vi "Combine Frame Data.vi"(7 "Block Diagram":T3, 10 "Frames-Owners":T5(array[cluster]), 11 "Frames Array":T4(array[cluster])) -> (3 "Frame Data":T2(array[cluster]))   [LabVIEW 2026]
doc: "This VI takes in the array of Frames and the array mapping the frames to their owners and combines them, returning an array of clusters that contain the data from the frame array and the owner uid for each frame."
uses:
  <vilib>/picture/picture.llb/imagedata.ctl
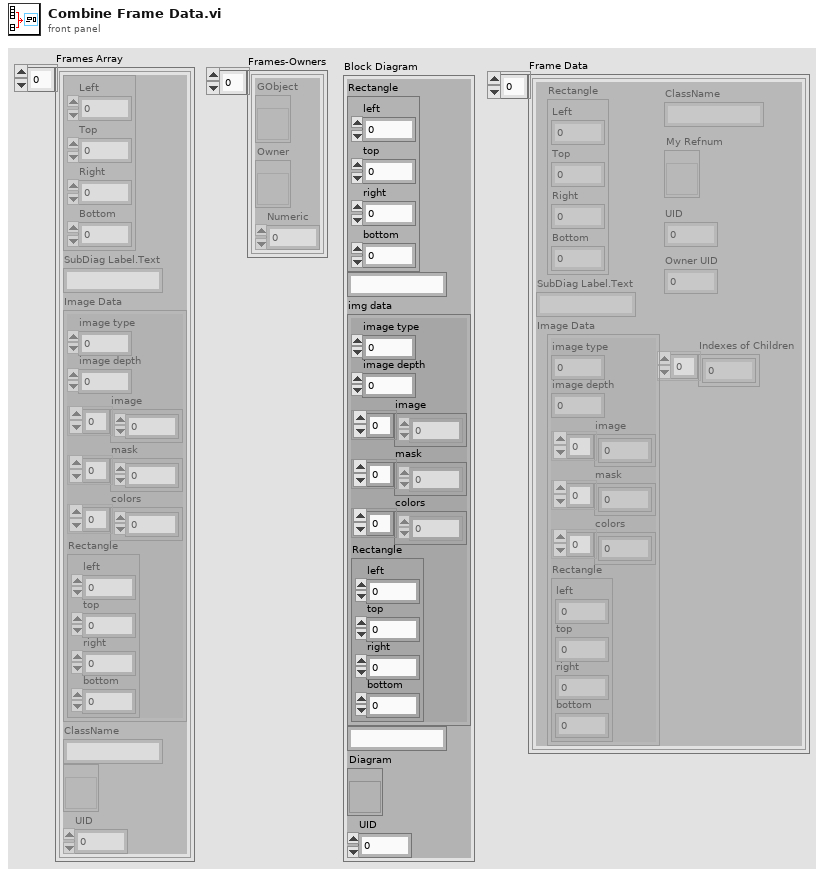
[diagram p1: front panel]
types:
  T1 = typedef "imagedata.ctl" = cluster{"image type":i32, "image depth":i32, "image":u8[], "mask":u8[], "colors":u32[], "Rectangle":cluster{"left":i16, "top":i16, "right":i16, "bottom":i16}}
  T2 = cluster{"Rectangle":cluster{"Left":i32, "Top":i32, "Right":u32, "Bottom":u32}, "SubDiag Label.Text":string, "Image Data":T1, "ClassName":string, "My Refnum":refnum<vi>, "UID":i32, "Owner UID":i32, "Indexes of Children":i32[]}[]
  T3 = cluster{"Rectangle":cluster{"left":i16, "top":i16, "right":i16, "bottom":i16}, string, "img data":T1, string, "Diagram":refnum<vi>, "UID":i32}
  T4 = cluster{cluster{"Left":i32, "Top":i32, "Right":u32, "Bottom":u32}, "SubDiag Label.Text":string, "Image Data":T1, "ClassName":string, refnum<vi>, "UID":i32}[]
  T5 = cluster{"GObject":refnum<vi>, "Owner":refnum<vi>, "Numeric":dbl}[]
  T6 = cluster{"Rectangle":cluster{"Left":i32, "Top":i32, "Right":u32, "Bottom":u32}, "SubDiag Label.Text":string, "Image Data":T1, "ClassName":string, "My Refnum":refnum<vi>, "UID":i32, "Owner UID":i32}[]
  T7 = cluster{cluster{"Left":i32, "Top":i32, "Right":u32, "Bottom":u32}, "SubDiag Label.Text":string, "Image Data":T1, "ClassName":string, refnum<vi>, "UID":i32, "UID":i32}
  T8 = cluster{"Left":i32, "Top":i32, "Right":u32, "Bottom":u32}
  T9 = cluster{cluster{"Left":i32, "Top":i32, "Right":u32, "Bottom":u32}, "SubDiag Label.Text":string, "Image Data":T1, "ClassName":string, refnum<vi>, "UID":i32, "Numeric":dbl}
  T10 = cluster{"Rectangle":cluster{"Left":i32, "Top":i32, "Right":u32, "Bottom":u32}, "SubDiag Label.Text":string, "Image Data":T1, "ClassName":string, "My Refnum":refnum<vi>, "UID":i32, "Owner UID":i32, i32[]}
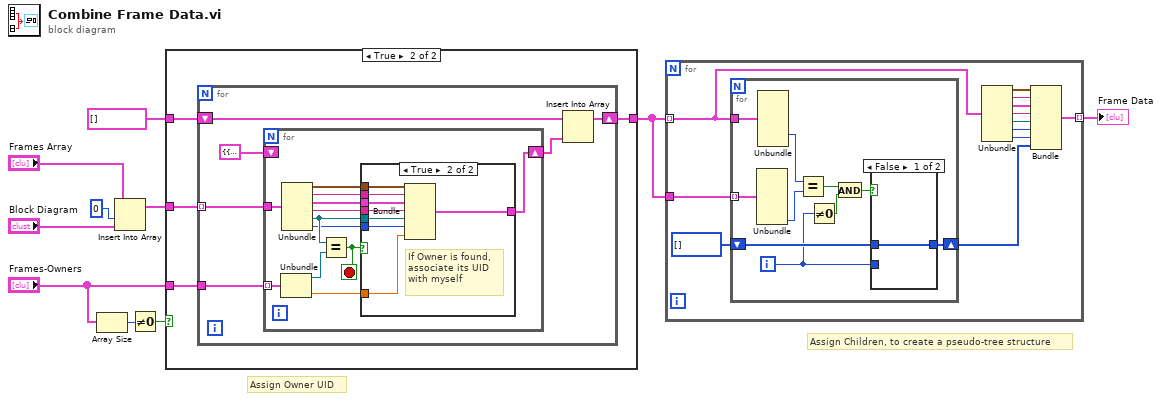
[diagram p0: block diagram]
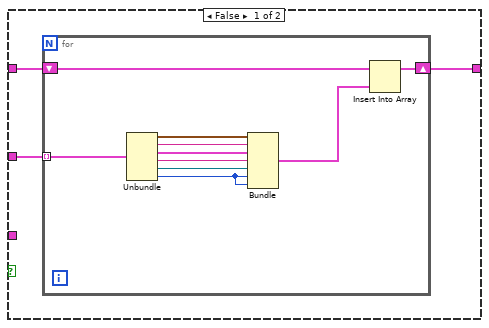
[diagram p2: hidden frame]
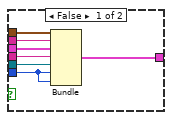
[diagram p3: hidden frame]
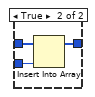
[diagram p4: hidden frame]
diagram:
  # "Assign Children, to create a pseudo-tree structure"
  # "Assign Owner UID"
  n1 = Array Size(array="Frames-Owners") -> (size(s)=w5:i32)
  n2 = Insert Into Array(array="Frames Array", index=0, new element="Block Diagram") -> (w8:T4)
  n3 = Not Equal To 0?(x=w5) -> (x != 0?=w6:bool)
  n4 = case shown="True" w6 {
    tunnel: w8 -> [w13 w27]
    tunnel: "Frames-Owners" -> [_ w26]
    tunnel: [w11 w25] -> w2
    tunnel: T6 [] -> [w12 w24]
    frame False {
      n5 = for {
        tunnel: w13 -> [w23] mode=indexing
        shift-right: [w21] -> w11
        shift-left: w12 -> [w22]
        n6 = Unbundle(w23) -> (w19:T8, "SubDiag Label.Text"=w18:string, "Image Data"=w17:T1, "ClassName"=w16:string, w15:refnum<vi>, "UID"=w14:i32)
        n7 = Bundle(w19, "SubDiag Label.Text"=w18, "Image Data"=w17, "ClassName"=w16, w15, "UID"=w14, "UID"=w14) -> (w20:T7)  [unwired: 1 in]
        n8 = Insert Into Array(array=w22, new element=w20) -> (w21:T6)  [unwired: 1 in]
      }
    }
    frame True {
      n9 = for {
        tunnel: w27 -> [w32] mode=indexing
        tunnel: w26 -> [w33]
        shift-right: [w30] -> w25
        shift-left: w24 -> [w31]
        n10 = for {
          tunnel: w33 -> [w44] mode=indexing
          tunnel: w32 -> [w45]
          shift-right: [w34] -> w28
          shift-left: T7 {{"Left"=0, "Top"=0, "Right"=0, "Bottom"=0}, "SubDiag Label.Text"="", "Image Data"={"image type"=0, "image depth"=0, "image"=[], "mask"=[], "colors"=[], "Rectangle"={"left"=0, "top"=0, "right"=0, "bottom"=0}}, "ClassName"="", refnum, "UID"=0, "UID"=0} ("output cluster") -> [_]
          stop <- w35 stop-if-true
          n11 = Unbundle(w44) -> ("GObject"=w43:refnum<vi>, "Numeric"=w36:dbl)  [unwired: 1 out]
          n12 = Unbundle(w45) -> (w42:T8, "SubDiag Label.Text"=w41:string, "Image Data"=w40:T1, "ClassName"=w39:string, w38:refnum<vi>, "UID"=w37:i32)
          n13 = Equal?(x=w38, y=w43) -> (x = y?=w35:bool)
          n14 = case shown="True" w35 {
            tunnel: w42 -> [w52 w60]
            tunnel: w41 -> [w51 w59]
            tunnel: w40 -> [w50 w58]
            tunnel: w39 -> [w49 w57]
            tunnel: w38 -> [w48 w56]
            tunnel: w37 -> [w47 w55]
            tunnel: w36 -> [_ w54]
            tunnel: [w46 w53] -> w34
            frame False {
              n15 = Bundle(w52, "SubDiag Label.Text"=w51, "Image Data"=w50, "ClassName"=w49, w48, "UID"=w47, "UID"=w47) -> (w46:T7)  [unwired: 1 in]
            }
            frame True {
              # "If Owner is found,\nassociate its UID\nwith myself"
              n16 = Bundle(w60, "SubDiag Label.Text"=w59, "Image Data"=w58, "ClassName"=w57, w56, "UID"=w55, "Numeric"=w54) -> (w53:T9)  [unwired: 1 in]
            }
          }
        }
        n17 = Insert Into Array(array=w31, new element=w28) -> (w30:T6)  [unwired: 1 in]
      }
    }
  }
  n18 = for {
    tunnel: w2 -> [w70] mode=indexing
    tunnel: w2 -> [w72]
    tunnel: [w61] -> w1 mode=indexing
    n19 = for {
      tunnel: w70 -> [w82]
      tunnel: w72 -> [w81] mode=indexing
      shift-right: [w77] -> w62
      shift-left: i32[] [] -> [w78]
      i -> [w73]
      n20 = Unbundle(w81) -> ("Owner UID"=w79:i32)  [unwired: 6 out]
      n21 = Unbundle(w82) -> ("UID"=w80:i32)  [unwired: 6 out]
      n22 = Equal?(x=w80, y=w79) -> (x = y?=w76:bool)
      n23 = Not Equal To 0?(x=w73) -> (x != 0?=w74:bool)
      n24 = And(x=w76, y=w74) -> (x .and. y?=w75:bool)
      n25 = case shown="False" w75 {
        tunnel: w78 -> [w83 w86]
        tunnel: [w83 w85] -> w77
        tunnel: w73 -> [_ w84]
        frame False {
        }
        frame True {
          n26 = Insert Into Array(array=w86, new element=w84) -> (w85:i32[])  [unwired: 1 in]
        }
      }
    }
    n27 = Unbundle(w70) -> ("Rectangle"=w68:T8, "SubDiag Label.Text"=w69:string, "Image Data"=w67:T1, "ClassName"=w66:string, "My Refnum"=w65:refnum<vi>, "UID"=w64:i32, "Owner UID"=w63:i32)
    n28 = Bundle("Rectangle"=w68, "SubDiag Label.Text"=w69, "Image Data"=w67, "ClassName"=w66, "My Refnum"=w65, "UID"=w64, "Owner UID"=w63, w62) -> (w61:T10)  [unwired: 1 in]
  }
  "Frame Data" <- w1
